vi "Values (I32).vi"(11 "Dictionary in":variant) -> (1 "Values":i32[](array[numeric]), 3 "Dictionary out":variant)   [LabVIEW 2013, in "Dictionary.lvlib"]
doc: "Returns all values in the dictionary."
uses:
  Dictionary.lvlib
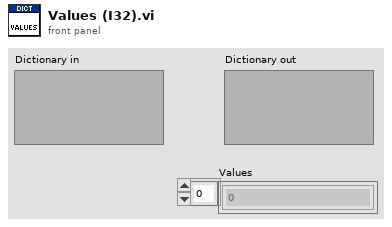
[diagram p1: front panel]
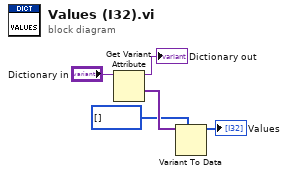
[diagram p0: block diagram]
diagram:
  n1 = Get Variant Attribute(Variant="Dictionary in") -> (duplicate Variant=→"Dictionary out":variant, values=w3:variant[])  [unwired: 3 in, 2 out]
  n2 = Variant To Data(type=i32[] [], Variant=w3) -> (data=→"Values":i32[])  [unwired: 1 in, 1 out]
